vi "Tosca-Update AO Frame Triggers.vi"(0 "Tosca":refnum<class "Parameters.lvclass">, 11 "error in (no error)":errorcluster) -> (4 "Tosca out":refnum<class "Parameters.lvclass">, 15 "error out":errorcluster)   [LabVIEW 2020]
uses:
  Classes/Parameters/Parameters.lvclass
  Tosca-Imaging Mode.ctl
  epl-vi-lib/Signal Synthesis VIs/4th Generation/Classes/Level/LevelUnits.ctl
  epl-vi-lib/Signal Synthesis VIs/4th Generation/Classes/Level/Level.lvclass/Level.ctl
  Classes/Parameters/Parameters.lvclass/Parameters.ctl
  epl-vi-lib/Signal Synthesis VIs/4th Generation/Classes/Waveforms/Pulse Train/Pulse Train.lvclass/Pulse Train.ctl
  Classes/State/State.lvclass/State.ctl
  epl-vi-lib/Signal Synthesis VIs/4th Generation/Classes/Channel/Channel.lvclass/Channel.ctl
  epl-vi-lib/Signal Synthesis VIs/4th Generation/Classes/Channel/Write Destination.vi
  epl-vi-lib/Signal Synthesis VIs/4th Generation/Classes/Channel/Write Waveform.vi
  epl-vi-lib/Signal Synthesis VIs/4th Generation/Classes/Channel/Write Level.vi
  epl-vi-lib/Signal Synthesis VIs/4th Generation/Classes/Channel/Write Persist.vi
  Classes/State/Read SigMan.vi
  Classes/State/Write SigMan.vi
  epl-vi-lib/Signal Synthesis VIs/4th Generation/Classes/Level/Write Units.vi
  epl-vi-lib/Signal Synthesis VIs/4th Generation/Classes/Level/Write Level.vi
  Classes/Parameters/Read Imaging.vi
  epl-vi-lib/Signal Synthesis VIs/4th Generation/Classes/Waveforms/Pulse Train/Write Rate (Hz).vi
  Classes/Parameters/Read Flowchart.vi
  Classes/Parameters/Write Flowchart.vi
  epl-vi-lib/Signal Synthesis VIs/4th Generation/Classes/Waveforms/Pulse Train/Pulse Train.lvclass
  D:/Development/epl-vi-lib/Signal Synthesis VIs/4th Generation/Classes/Waveforms/Waveform/Waveform.lvclass
  Classes/State/State.lvclass
  epl-vi-lib/Signal Synthesis VIs/4th Generation/Classes/SignalManager/SignalManager.lvclass
  epl-vi-lib/Signal Synthesis VIs/4th Generation/Classes/Channel/Channel.lvclass
  epl-vi-lib/Signal Synthesis VIs/4th Generation/Classes/Level/Level.lvclass
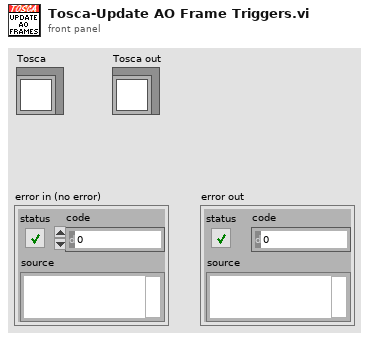
[diagram p1: front panel]
types:
  T1 = typedef "Level.lvclass/LevelUnits.ctl" = enum16{"dB atten", "dB SPL", "dB Vrms", "Volts", "dB mW", "mW", "dB HL", "dB SL"}
  T2 = typedef "Tosca-Imaging Mode.ctl" = enum16{"Off", "Widefield", "Two-photon"}
  T3 = typedef "Tosca-Imaging.ctl" = cluster{"mode":T2, "FrameRateHz":dbl, "use AO":bool, "destination":string}
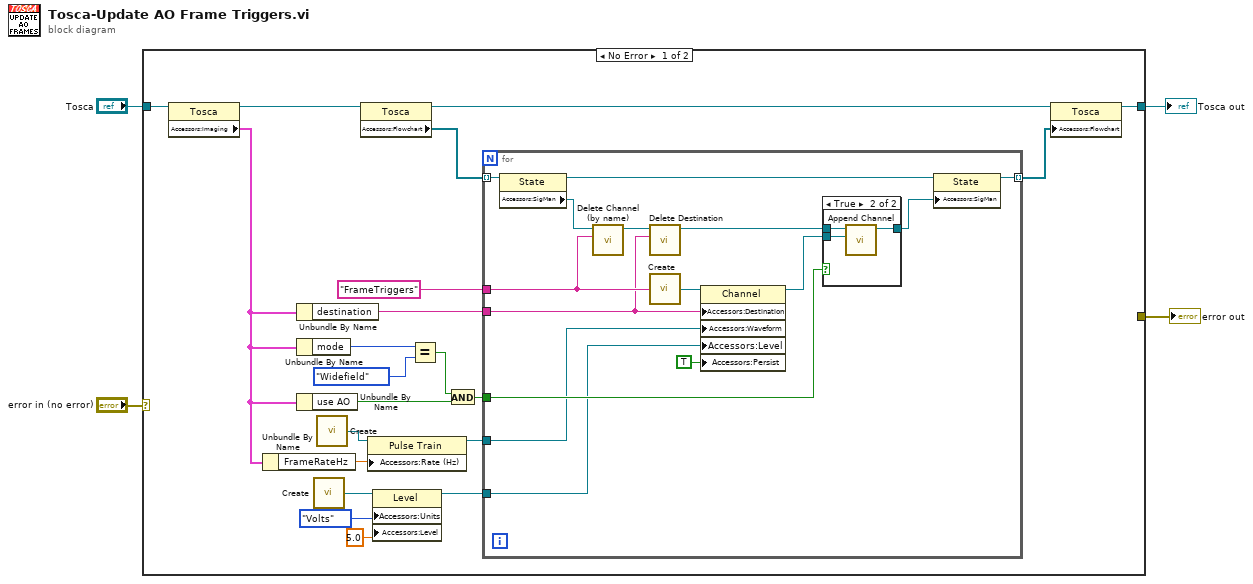
[diagram p0: block diagram]
diagram:
  n1 = case shown="No Error" "error in (no error)" {
    selector: "error in (no error)" -> [_ w45]
    tunnel: [_ w45] -> w3
    tunnel: [w18 w46] -> w1
    tunnel: "Tosca" -> [w24 w46]
    frame No Error {
      n2 = property class="Tosca"(reference=w24) -> (reference out=w20:refnum<class "Parameters.lvclass">, "Accessors:Imaging"=w10:T3)  [unwired: 1 in, 1 out]
      n3 = Unbundle By Name(w10) -> ("FrameRateHz"=w9:dbl)
      n4 = Unbundle By Name(w10) -> ("destination"=w17:string)
      n5 = Unbundle By Name(w10) -> ("mode"=w23:T2)
      n6 = Unbundle By Name(w10) -> ("use AO"=w21:bool)
      n7 = call "Create.vi"() -> ("Level"=w8:refnum<class "Level.lvclass">)  [unwired: 15 in]
      n8 = call "Create.vi"() -> ("Pulse Train"=w12:refnum<class "Pulse Train.lvclass">)  [unwired: 15 in]
      n9 = property class="Tosca"(reference=w20) -> (reference out=w15:refnum<class "Parameters.lvclass">, "Accessors:Flowchart"=w16:refnum<class "State.lvclass">[])  [unwired: 1 in, 1 out]
      n10 = property class="Pulse Train"(reference=w12, "Accessors:Rate (Hz)"=w9) -> (reference out=w11:refnum<class "Pulse Train.lvclass">)  [unwired: 1 in, 1 out]
      n11 = property class="Level"(reference=w8, "Accessors:Units"=LevelUnits."Volts" ("Units"), "Accessors:Level"=5.0 ("Level")) -> (reference out=w7:refnum<class "Level.lvclass">)  [unwired: 1 in, 1 out]
      n12 = Equal?(x=w23, y=Tosca-Imaging_Mode."Widefield") -> (x = y?=w22:bool)
      n13 = And(x=w22, y=w21) -> (x .and. y?=w13:bool)
      n14 = for {
        tunnel: w16 -> [w40] mode=indexing
        tunnel: "FrameTriggers" -> [w36]
        tunnel: [w28] -> w14 mode=indexing
        tunnel: w17 -> [w32]
        tunnel: w13 -> [w29]
        tunnel: w11 -> [w27]
        tunnel: w7 -> [w26]
        n15 = property class="State"(reference=w40) -> (reference out=w39:refnum<class "State.lvclass">, "Accessors:SigMan"=w38:refnum<class "SignalManager.lvclass">)  [unwired: 1 in, 1 out]
        n16 = call "Delete Channel (by name).vi"("Name"=w36, "SigMan in"=w38) -> ("SigMan out"=w37:refnum<class "SignalManager.lvclass">)  [unwired: 8 in, 1 out]
        n17 = call "Delete Destination.vi"("Name"=w32, "SigMan in"=w37) -> ("SigMan out"=w35:refnum<class "SignalManager.lvclass">)  [unwired: 8 in, 1 out]
        n18 = call "Create.vi"("Name"=w36) -> ("Channel"=w33:refnum<class "Channel.lvclass">)  [unwired: 14 in]
        n19 = property class="Channel"(reference=w33, "Accessors:Destination"=w32, "Accessors:Waveform"=w27, "Accessors:Level"=w26, "Accessors:Persist"=TRUE ("Persist")) -> (reference out=w31:refnum<class "Channel.lvclass">)  [unwired: 1 in, 1 out]
        n20 = case shown="True" w29 {
          tunnel: w35 -> [w41 w44]
          tunnel: [w41 w43] -> w34
          tunnel: w31 -> [_ w42]
          frame False {
          }
          frame True {
            n21 = call "Append Channel.vi"("Channel"=w42, "SignalManager in"=w44) -> ("SignalManager out"=w43:refnum<class "SignalManager.lvclass">)  [unwired: 8 in, 1 out]
          }
        }
        n22 = property class="State"(reference=w39, "Accessors:SigMan"=w34) -> (reference out=w28:refnum<class "State.lvclass">)  [unwired: 1 in, 1 out]
      }
      n23 = property class="Tosca"(reference=w15, "Accessors:Flowchart"=w14) -> (reference out=w18:refnum<class "Parameters.lvclass">)  [unwired: 1 in, 1 out]
    }
    frame Error {
    }
  }
  "Tosca out" <- w1
  "error out" <- w3
